vi "Viewport Sizes.vi"() -> (0 "Viewport Size y/2":i32, 1 "Viewport Size y":i32, 2 "Viewport Size x/2":i32, 3 "Viewport Size x":i32, 4 "Viewport Size y*2":i32, 5 "Viewport Size x*2":i32)   [LabVIEW 2015]
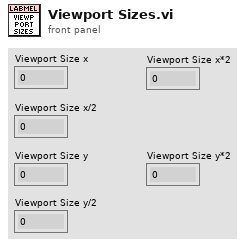
[diagram p1: front panel]
types:
  T1 = typedef "Constants.ctl" = cluster{"Colours":cluster{"OK":u32, "Warning":u32, "Error":u32, "Red":u32, "Green":u32, "Blue":u32, "Yellow":u32}, "System":cluster{"Target Frames Second":dbl, "Field Size":T2, "Window Size":T2, "Viewport Size":T2, "Sidebar Scaling":sgl, "Sidebar Width":i32}, "Game":cluster{"Maximum Asteroids":i32, "Max Energy":i32, "Max Crew":i32}}
  T2 = typedef "SDL2 Utility.lvlib/Point (I32).ctl" = cluster{"x":i32, "y":i32}
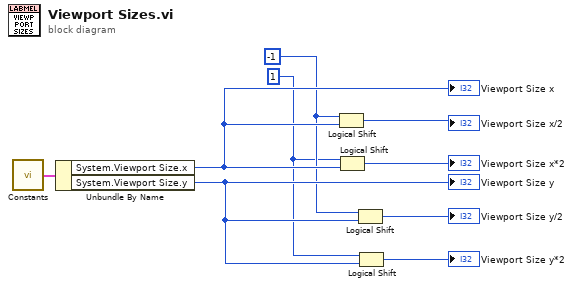
[diagram p0: block diagram]
diagram:
  w3 = i16 1 ("y")
  w4 = i16 -1 ("y")
  n1 = call "Constants.vi"() -> ("Constants"=w9:T1)
  n2 = Unbundle By Name(w9) -> ("System.Viewport Size.x"=w7:i32, "System.Viewport Size.y"=w5:i32)
  "Viewport Size x" <- w7
  "Viewport Size y" <- w5
  n3 = Logical Shift(y=w4, x=w7) -> (x << y=→"Viewport Size x/2":i32)
  n4 = Logical Shift(y=w3, x=w7) -> (x << y=→"Viewport Size x*2":i32)
  n5 = Logical Shift(y=w4, x=w5) -> (x << y=→"Viewport Size y/2":i32)
  n6 = Logical Shift(y=w3, x=w5) -> (x << y=→"Viewport Size y*2":i32)
